vi "SensorColorSubVI2.vi"(0 "Frecuencia 1":bool=TRUE, 1 "Frecuencia in":bool) -> (2 "Sin Filtro":dbl format="%.2f", 3 "Rojo":dbl format="%.2f", 4 "Verde":dbl format="%.2f", 5 "Azul":dbl)   [LabVIEW 2017]
uses:
  enumColor.ctl
  <vilib>/DAQmx/write.llb/DAQmx Write (Digital 1D Bool 1Chan 1Samp).vi
  <vilib>/DAQmx/read.llb/DAQmx Read (Counter DBL 1Chan 1Samp).vi
  <vilib>/DAQmx/create/channels.llb/DAQmx Create Channel (DO-Digital Output).vi
  <vilib>/DAQmx/create/channels.llb/DAQmx Create Channel (CI-Count Edges).vi
  <vilib>/DAQmx/miscellaneous.llb/DAQmx Fill In Error Info.vi
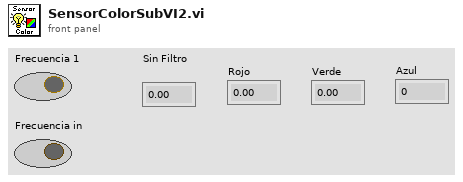
[diagram p1: front panel]
types:
  T1 = typedef "enumColor.ctl" = enum16{"Inicio", "SinFiltro1", "SinFiltro2", "SinFiltro3", "Rojo1", "Rojo2", "Rojo3", "Verde1", "Verde2", "Verde3", "Azul1", "Azul2", "Azul3", "Cierre"}
  T2 = cluster{"task out":refnum<k21>, "error out":errorcluster}
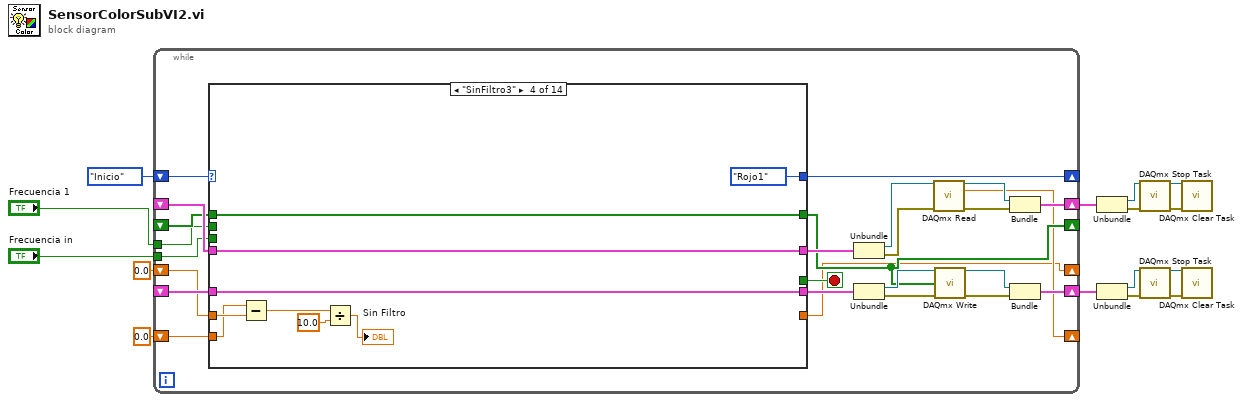
[diagram p0: block diagram]
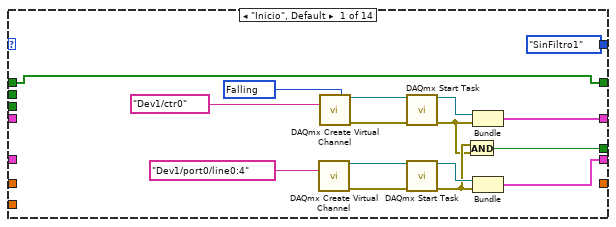
[diagram p2: hidden frame]
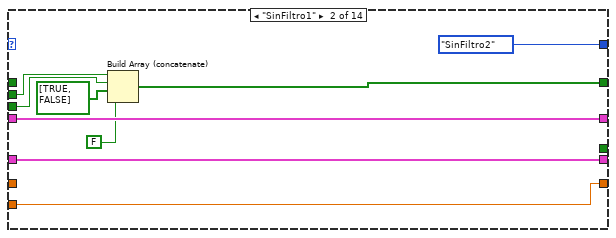
[diagram p3: hidden frame]
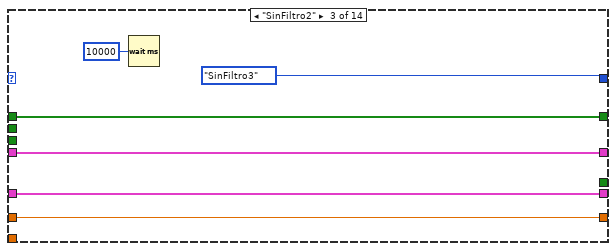
[diagram p4: hidden frame]
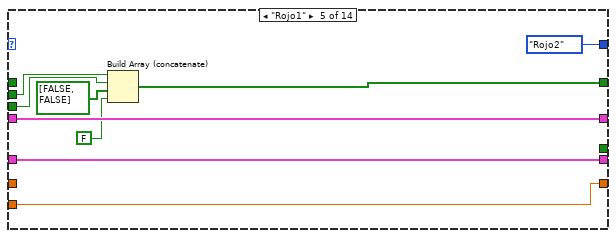
[diagram p5: hidden frame]
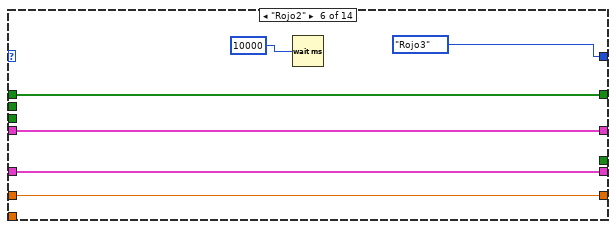
[diagram p6: hidden frame]
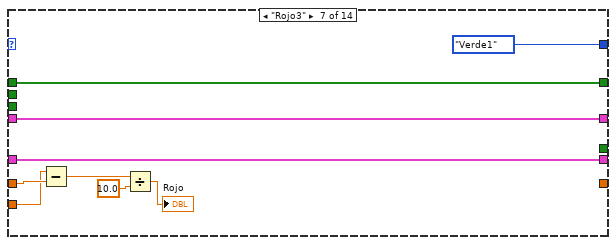
[diagram p7: hidden frame]
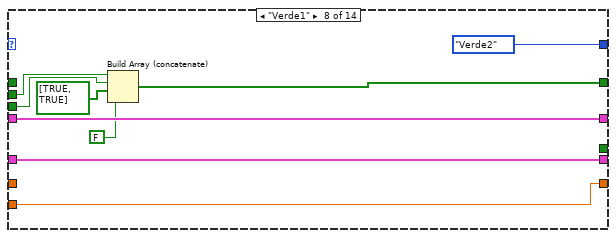
[diagram p8: hidden frame]
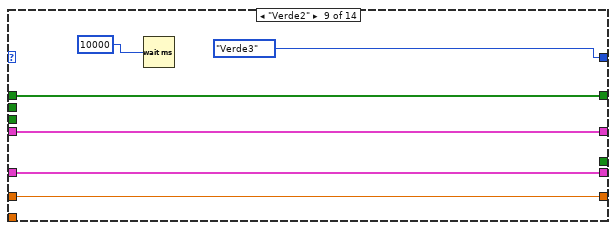
[diagram p9: hidden frame]
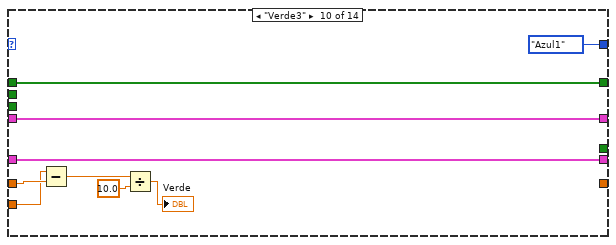
[diagram p10: hidden frame]
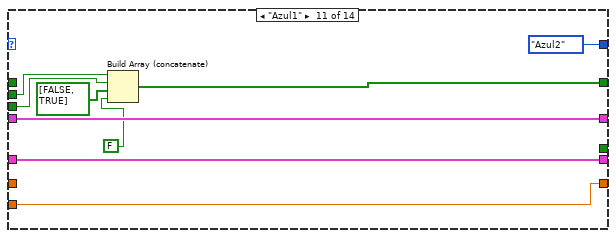
[diagram p11: hidden frame]
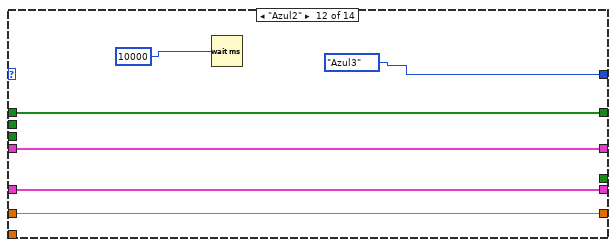
[diagram p12: hidden frame]
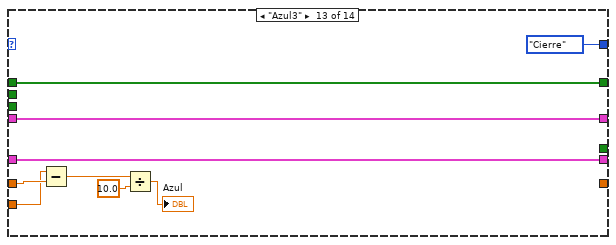
[diagram p13: hidden frame]
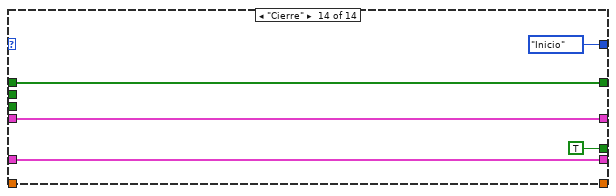
[diagram p14: hidden frame]
diagram:
  n1 = while {
    shift-right: [w39] -> _
    shift-left: enumColor."Inicio" -> [w24]
    shift-right: [w25] -> w13
    shift-left: _ -> [w26]
    shift-right: [w33] -> w12
    shift-left: _ -> [w30]
    tunnel: "Frecuencia 1" -> [w16]
    tunnel: "Frecuencia in" -> [w17]
    shift-right: [w23] -> _
    shift-left: _ -> [w22]
    shift-right: [w21] -> _
    shift-left: 0.0 ("data") -> [w20]
    shift-right: [w19] -> _
    shift-left: 0.0 ("data") -> [w18]
    stop <- w40 stop-if-true
    n2 = case shown="\"SinFiltro3\"" w24 {
      tunnel: [w52 _ _ _ _ _ _ _ _ _ _ _ _ TRUE] -> w40
      tunnel: [w46 w65 w71 w80 w85 w95 w103 w108 w119 w127 w132 w143 w151 w156] -> w36
      tunnel: [enumColor."SinFiltro1" enumColor."SinFiltro2" enumColor."SinFiltro3" enumColor."Rojo1" enumColor."Rojo2" enumColor."Rojo3" enumColor."Verde1" enumColor."Verde2" enumColor."Verde3" enumColor."Azul1" enumColor."Azul2" enumColor."Azul3" enumColor."Cierre" enumColor."Inicio"] -> w39
      tunnel: w16 -> [_ w62 _ _ w88 _ _ w112 _ _ w136 _ _ _]
      tunnel: w17 -> [_ w61 _ _ w87 _ _ w111 _ _ w135 _ _ _]
      tunnel: [w43 w60 w70 w79 w86 w93 w102 w110 w117 w126 w134 w141 w150 w153] -> w23
      tunnel: w30 -> [_ w65 w71 w80 w85 w95 w103 w108 w119 w127 w132 w143 w151 w156]
      tunnel: [w44 w64 w69 w78 w84 w94 w104 w109 w118 w128 w133 w142 w152 w157] -> w27
      tunnel: w26 -> [_ w64 w69 w78 w84 w94 w104 w109 w118 w128 w133 w142 w152 w157]
      tunnel: w22 -> [w43 _ w70 w79 _ w93 w102 _ w117 w126 _ w141 w150 w153]
      tunnel: w20 -> [_ w58 _ w72 w82 _ w96 w106 _ w120 w131 _ w144 _]
      tunnel: [_ w58 w68 _ w82 w92 _ w106 w116 _ w131 w140 _ _] -> w19
      tunnel: w18 -> [_ _ w68 w74 _ w92 w101 _ w116 w125 _ w140 w147 _]
      frame "Inicio", Default {
        w41 = 10171 items=["Rising"=10280, "Falling"=10171] ("edge")
        n3 = call-poly <vilib>:"DAQmx Create Virtual Channel.vi"("lines"=tag "Dev1/port0/line0:4") -> ("task out"=w56:refnum<k21>, "error out"=w55:errorcluster)  [unwired: 13 in]
        n4 = call-poly <vilib>:"DAQmx Create Virtual Channel.vi"("edge"=w41, "counter"=tag "Dev1/ctr0") -> ("task out"=w54:refnum<k21>, "error out"=w53:errorcluster)  [unwired: 12 in]
        n5 = call <vilib>:"DAQmx Start Task.vi"("task/channels in"=w54, "error in"=w53) -> ("task out"=w48:refnum<k21>, "error out"=w47:errorcluster)  [unwired: 12 in]
        n6 = call <vilib>:"DAQmx Start Task.vi"("task/channels in"=w56, "error in"=w55) -> ("task out"=w50:refnum<k21>, "error out"=w49:errorcluster)  [unwired: 12 in]
        n7 = And(x=w49, y=w47) -> (x .and. y?=w52:bool)
        n8 = Bundle("task out"=w48, "error out"=w47) -> (w46:T2)  [unwired: 1 in]
        n9 = Bundle("task out"=w50, "error out"=w49) -> (w44:T2)  [unwired: 1 in]
      }
      frame "SinFiltro1" {
        n10 = Build Array (concatenate)(w62, w61, bool[] [TRUE, FALSE], FALSE) -> (w60:bool[])
      }
      frame "SinFiltro2" {
        n11 = Wait (ms)(milliseconds to wait=u32 10000) -> ()  [unwired: 1 out]
      }
      frame "SinFiltro3" {
        n12 = Subtract(x=w72, y=w74) -> (x-y=w77:dbl)
        n13 = Divide(x=w77, y=10.0) -> (x/y=→"Sin Filtro":dbl)
      }
      frame "Rojo1" {
        n14 = Build Array (concatenate)(w88, w87, bool[] [FALSE, FALSE], FALSE) -> (w86:bool[])
      }
      frame "Rojo2" {
        n15 = Wait (ms)(milliseconds to wait=u32 10000) -> ()  [unwired: 1 out]
      }
      frame "Rojo3" {
        n16 = Subtract(x=w96, y=w101) -> (x-y=w100:dbl)
        n17 = Divide(x=w100, y=10.0) -> (x/y=→"Rojo":dbl)
      }
      frame "Verde1" {
        n18 = Build Array (concatenate)(w112, w111, bool[] [TRUE, TRUE], FALSE) -> (w110:bool[])
      }
      frame "Verde2" {
        n19 = Wait (ms)(milliseconds to wait=u32 10000 ("millisecond timer value")) -> ()  [unwired: 1 out]
      }
      frame "Verde3" {
        n20 = Subtract(x=w120, y=w125) -> (x-y=w123:dbl)
        n21 = Divide(x=w123, y=10.0 ("x")) -> (x/y=→"Verde":dbl)
      }
      frame "Azul1" {
        n22 = Build Array (concatenate)(w136, w135, bool[] [FALSE, TRUE], FALSE) -> (w134:bool[])
      }
      frame "Azul2" {
        n23 = Wait (ms)(milliseconds to wait=u32 10000 ("millisecond timer value")) -> ()  [unwired: 1 out]
      }
      frame "Azul3" {
        n24 = Subtract(x=w144, y=w147) -> (x-y=w148:dbl)
        n25 = Divide(x=w148, y=10.0) -> (x/y=→"Azul":dbl)
      }
      frame "Cierre" {
      }
    }
    n26 = Unbundle(w36) -> ("task out"=w35:refnum<k21>, "error out"=w34:errorcluster)
    n27 = Unbundle(w27) -> ("task out"=w38:refnum<k21>, "error out"=w37:errorcluster)
    n28 = call-poly <vilib>:"DAQmx Read.vi"("task/channels in"=w35, "error in"=w34) -> ("task out"=w32:refnum<k21>, "data"=w21:dbl, "error out"=w31:errorcluster)  [unwired: 11 in]
    n29 = call-poly <vilib>:"DAQmx Write.vi"("task/channels in"=w38, "data"=w23, "error in"=w37) -> ("task out"=w29:refnum<k21>, "error out"=w28:errorcluster)  [unwired: 10 in, 1 out]
    n30 = Bundle("task out"=w32, "error out"=w31) -> (w33:T2)  [unwired: 1 in]
    n31 = Bundle("task out"=w29, "error out"=w28) -> (w25:T2)  [unwired: 1 in]
  }
  n32 = Unbundle(w12) -> ("task out"=w9:refnum<k21>, "error out"=w8:errorcluster)
  n33 = Unbundle(w13) -> ("task out"=w11:refnum<k21>, "error out"=w10:errorcluster)
  n34 = call <vilib>:"DAQmx Stop Task.vi"("task/channels in"=w9, "error in"=w8) -> ("task out"=w5:refnum<k21>, "error out"=w4:errorcluster)  [unwired: 12 in]
  n35 = call <vilib>:"DAQmx Stop Task.vi"("task/channels in"=w11, "error in"=w10) -> ("task out"=w7:refnum<k21>, "error out"=w6:errorcluster)  [unwired: 12 in]
  n36 = call <vilib>:"DAQmx Clear Task.vi"("task in"=w5, "error in"=w4) -> ()  [unwired: 13 in, 1 out]
  n37 = call <vilib>:"DAQmx Clear Task.vi"("task in"=w7, "error in"=w6) -> ()  [unwired: 13 in, 1 out]
